vi "mtg reader - globals.vi"() -> ()   [LabVIEW 2025]
panel:
  in  "chunk size":i32=3
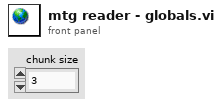
[diagram p1: front panel]
diagram:
